vi "SL_Facade.vi"(0 "Data In":T4, 2 "Display State In":T2, 3 "Container State":T3) -> (6 "Data Out":T4, 7 "Display State Out":T2, 8 "Action":T1)   [LabVIEW 2020, in "SL_XControl.xctl"]
uses:
  SL_XControl.xctl
  SL_Data.ctl
  <vilib>/_xctls/Container State.ctl
  SL_State.ctl
  <vilib>/_xctls/Action.ctl
  <vilib>/_xctls/XControlSupport.lvlib
panel:
  out "type":string
  out "value":string
  out "Toggle":bool
  out "info":string
  in  "Refresh":bool
  in  "Login":bool
  in  "Edit":bool
  in  "Property":string
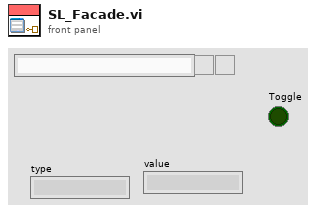
[diagram p1: front panel]
types:
  T1 = typedef "XControlSupport.lvlib/Action.ctl" = cluster{"Data Changed?":bool, "State Changed?":bool, "Action Name":string}
  T2 = typedef "SL_XControl.xctl/SL_State.ctl" = cluster{"Numeric":dbl}
  T3 = typedef "XControlSupport.lvlib/Container State.ctl" = cluster{"Indicator?":bool, "Run Mode?":bool, " Refnum":refnum<vi>}
  T4 = typedef "SL_XControl.xctl/SL_Data.ctl" = string
  T5 = enum8{"Enabled", "Disabled", "Disabled and Grayed Out"}
  T6 = cluster{"Name":string, "BaseURL":string, "AppKey":string, "Headers":string[], "Timeout":i32}
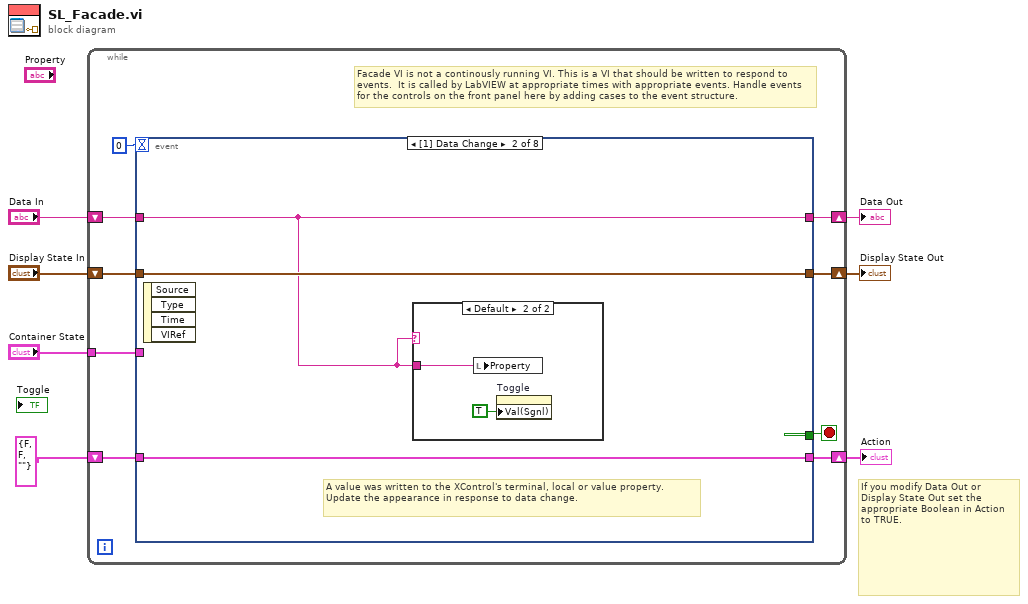
[diagram p0: block diagram]
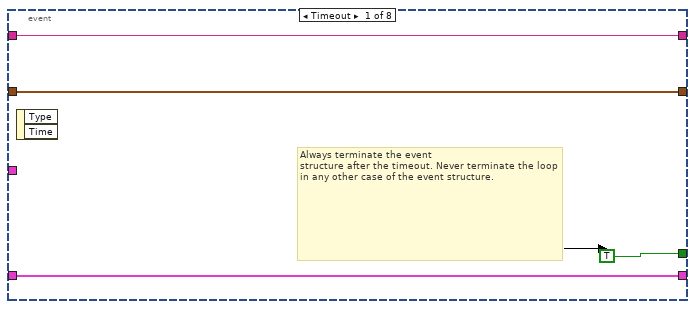
[diagram p2: hidden frame]
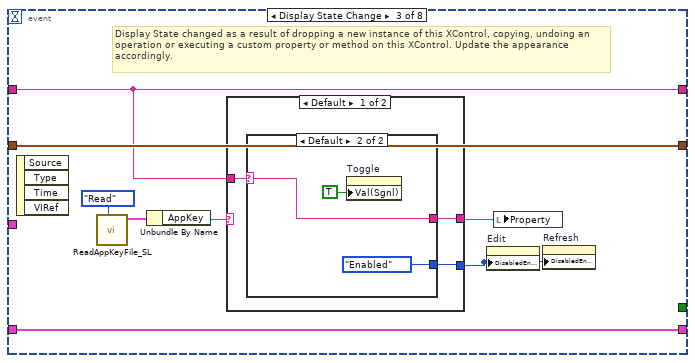
[diagram p4: hidden frame]
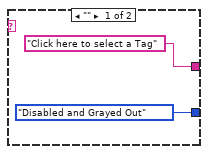
[diagram p5: hidden frame]
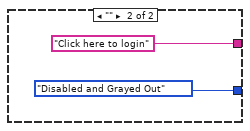
[diagram p6: hidden frame]
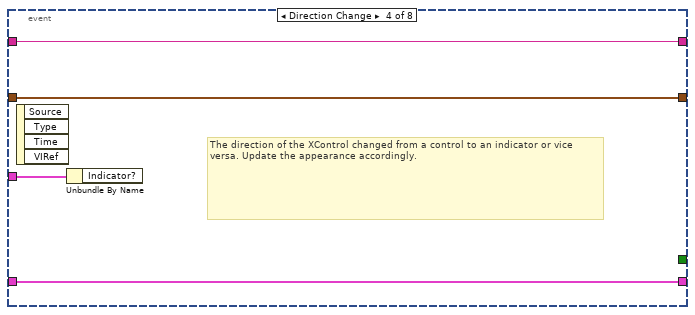
[diagram p7: hidden frame]
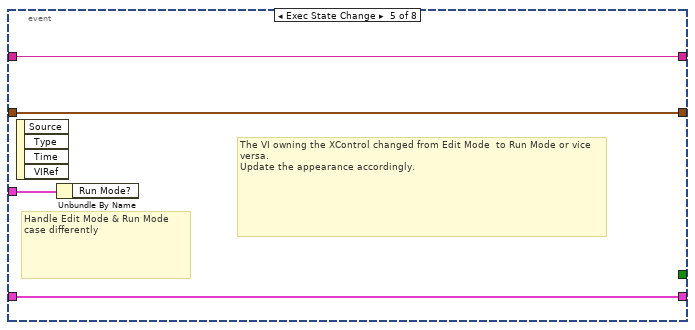
[diagram p8: hidden frame]
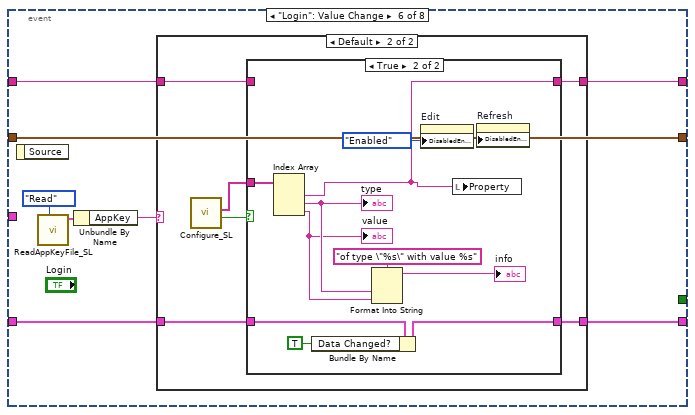
[diagram p9: hidden frame]
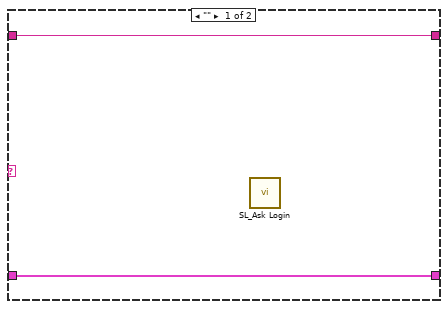
[diagram p10: hidden frame]
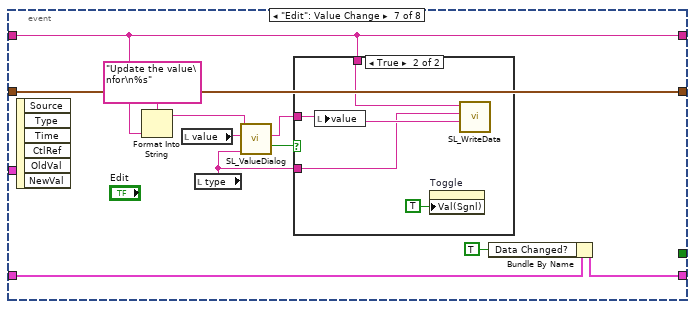
[diagram p12: hidden frame]
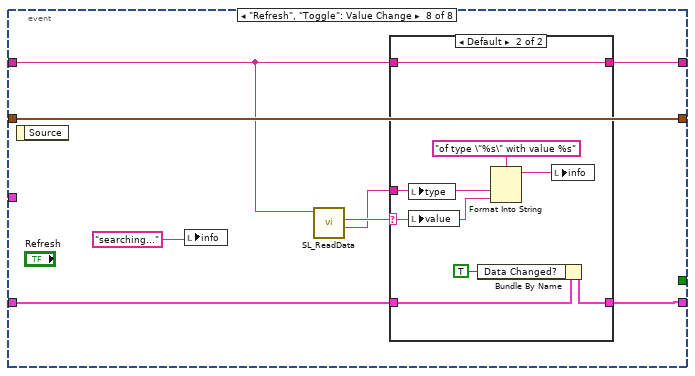
[diagram p14: hidden frame]
diagram:
  # "If you modify Data Out or\nDisplay State Out set the\nappropriate Boolean in Action\nto TRUE."
  n1 = while {
    shift-right: [w15] -> w4
    shift-left: "Display State In" -> [w16]
    tunnel: "Container State" -> [w12]
    shift-right: [w10] -> w7
    shift-left: "Data In" -> [w11]
    shift-right: [w8] -> w2
    shift-left: T1 {"Data Changed?"=FALSE, "State Changed?"=FALSE, "Action Name"=""} ("Action") -> [w9]
    stop <- w14 stop-if-true
    # "Facade VI is not a continously running VI. This is a VI that should be written to respond to events.  It is called by LabVIEW at appropriate times with appropriate events. Handle events for the controls on the front panel here by adding cases to the event structure."
    n2 = event shown="[1] Data Change" {
      selector: _ -> [_ _ _ _ _ _ _ _]
      dyn-events: _ -> [_ _ _ _ _ _ _ _]
      timeout: 0 -> [_ _ _ _ _ _ _ _]
      tunnel: w16 -> [w18 w23 w33 w46 w50 w59 w90 w102]
      tunnel: [w18 w23 w33 w46 w50 w59 w90 w102] -> w15
      tunnel: [TRUE _ _ _ _ _ _ _] -> w14
      tunnel: w12 -> [_ _ _ w47 w51 _ _ _]
      tunnel: w11 -> [w17 w21 w26 w45 w49 w56 w85 w95]
      tunnel: [w17 w21 w26 w45 w49 w55 w85 w101] -> w10
      tunnel: [w19 w22 w32 w44 w48 w57 w81 w99] -> w8
      tunnel: w9 -> [w19 w22 w32 w44 w48 w58 w82 w100]
      event Timeout {
        # "Always terminate the event\nstructure after the timeout. Never terminate the loop in any other case of the event structure."
        n3 = event-data() -> ()  [unwired: 1 in, 2 out]
      }
      event Data Change {
        # "A value was written to the XControl's terminal, local or value property.\nUpdate the appearance in response to data change."
        n4 = event-data() -> ()  [unwired: 1 in, 4 out]
        n5 = case shown="Default" w21 {
          tunnel: w21 -> [_ w24]
          frame "" {
          }
          frame Default {
            n6 = local write "Property"(w24) -> ()
            n7 = property on="Toggle" class="Bool (strict)"("Val(Sgnl)"=TRUE ("Value (Signaling)")) -> ()  [unwired: 2 in, 2 out]
          }
        }
      }
      event Display State Change {
        # "Display State changed as a result of dropping a new instance of this XControl, copying, undoing an operation or executing a custom property or method on this XControl. Update the appearance accordingly."
        n8 = event-data() -> ()  [unwired: 1 in, 4 out]
        n9 = call "ReadAppKeyFile_SL.vi"("Task"=enum16{"Read", "Write"}."Read") -> ("Device Out"=w31:T6)  [unwired: 8 in, 2 out]
        n10 = Unbundle By Name(w31) -> ("AppKey"=w30:string)
        n11 = case shown="Default" w30 {
          tunnel: [w36 "Click here to login" ("Property")] -> w29
          tunnel: [w35 T5."Disabled and Grayed Out" ("Disabled")] -> w28
          tunnel: w26 -> [w34 _]
          frame Default {
            n12 = case shown="Default" w34 {
              selector: w34 -> [_ w39]
              tunnel: ["Click here to select a Tag" ("Property") w39] -> w36
              tunnel: [T5."Disabled and Grayed Out" ("Disabled") T5."Enabled" ("Disabled")] -> w35
              frame "" {
              }
              frame Default {
                n13 = property on="Toggle" class="Bool (strict)"("Val(Sgnl)"=TRUE ("Value (Signaling)")) -> ()  [unwired: 2 in, 2 out]
              }
            }
          }
          frame "" {
          }
        }
        n14 = property on="Edit" class="Bool"("DisabledEnum"=w28) -> ()  [unwired: 2 in, 2 out]
        n15 = local write "Property"(w29) -> ()
        n16 = property on="Refresh" class="Bool"("DisabledEnum"=w28) -> ()  [unwired: 2 in, 2 out]
      }
      event Direction Change {
        # "The direction of the XControl changed from a control to an indicator or vice versa. Update the appearance accordingly."
        n17 = event-data() -> ()  [unwired: 1 in, 4 out]
        n18 = Unbundle By Name(w47) -> ()  [unwired: 1 out]
      }
      event Exec State Change {
        # "The VI owning the XControl changed from Edit Mode  to Run Mode or vice versa.\nUpdate the appearance accordingly."
        # "Handle Edit Mode & Run Mode\ncase differently"
        n19 = event-data() -> ()  [unwired: 1 in, 4 out]
        n20 = Unbundle By Name(w51) -> ()  [unwired: 1 out]
      }
      event "Login": Value Change {
        n21 = event-data() -> ()  [unwired: 1 in, 1 out]
        n22 = call "ReadAppKeyFile_SL.vi"("Task"=enum16{"Read", "Write"}."Read") -> ("Device Out"=w54:T6)  [unwired: 8 in, 2 out]
        n23 = Unbundle By Name(w54) -> ("AppKey"=w52:string)
        n24 = case shown="Default" w52 {
          tunnel: w58 -> [w60 w67]
          tunnel: [w60 w66] -> w57
          tunnel: w56 -> [w61 w65]
          tunnel: [w61 w64] -> w55
          frame "" {
            n25 = call "SL_Ask Login.vi"() -> ()  [unwired: 10 in, 2 out]
          }
          frame Default {
            n26 = call "Configure_SL.vi"() -> ("changed?"=w63:bool, "Property"=w62:string[])  [unwired: 10 in]
            n27 = case shown="True" w63 {
              tunnel: w65 -> [w69 _]
              tunnel: [w69 w72] -> w64
              tunnel: w62 -> [_ w79]
              tunnel: w67 -> [w68 w77]
              tunnel: [w68 w76] -> w66
              frame False {
              }
              frame True {
                w73 = T5."Enabled" ("Disabled")
                n28 = Index Array(array=w79) -> (element #1=w72:string, element #2=w71:string, element #3=w70:string)  [unwired: 3 in]
                "value" <- w70
                "type" <- w71
                n29 = Bundle By Name(cluster=w77, "Data Changed?"=TRUE) -> (w76:T1)
                n30 = Format Into String(format string="of type \"%s\" with value %s", w71, w70) -> (resulting string=→"info":string)  [unwired: 2 in, 1 out]
                n31 = property on="Edit" class="Bool"("DisabledEnum"=w73) -> ()  [unwired: 2 in, 2 out]
                n32 = local write "Property"(w72) -> ()
                n33 = property on="Refresh" class="Bool"("DisabledEnum"=w73) -> ()  [unwired: 2 in, 2 out]
              }
            }
          }
        }
      }
      event "Edit": Value Change {
        n34 = event-data() -> ()  [unwired: 1 in, 6 out]
        n35 = Format Into String(format string="Update the value\nfor\n%s", w85) -> (resulting string=w86:string)  [unwired: 2 in, 1 out]
        n36 = local read "value"() -> (w84:string)
        n37 = local read "type"() -> (w80:string)
        n38 = call "SL_ValueDialog.vi"("type"=w80, "Value"=w84, "Title"=w86) -> ("replace?"=w89:bool, "Value out"=w88:string)  [unwired: 7 in]
        n39 = case shown="True" w89 {
          tunnel: w85 -> [_ w93]
          tunnel: w88 -> [_ w92]
          tunnel: w80 -> [_ w91]
          frame False {
          }
          frame True {
            n40 = local write "value"(w92) -> ()
            n41 = property on="Toggle" class="Bool (strict)"("Val(Sgnl)"=TRUE ("Value (Signaling)")) -> ()  [unwired: 2 in, 2 out]
            n42 = call "SL_WriteData.vi"("Data"=w92, "Type"=w91, "Path"=w93) -> ()  [unwired: 9 in]
          }
        }
        n43 = Bundle By Name(cluster=w82, "Data Changed?"=TRUE) -> (w81:T1)
      }
      event "Refresh", "Toggle": Value Change {
        n44 = event-data() -> ()  [unwired: 1 in, 1 out]
        n45 = local write "info"("searching..." ("info")) -> ()
        n46 = call "SL_ReadData.vi"("Property"=w95) -> ("type"=w97:string, "value"=w98:string)  [unwired: 9 in]
        n47 = case shown="Default" w98 {
          selector: w98 -> [_ w106]
          tunnel: w95 -> [w104 w107]
          tunnel: [w104 w107] -> w101
          tunnel: w100 -> [w103 w112]
          tunnel: [w103 w111] -> w99
          tunnel: w97 -> [_ w105]
          frame "" {
          }
          frame Default {
            n48 = local write "type"(w105) -> ()
            n49 = local write "value"(w106) -> ()
            n50 = Bundle By Name(cluster=w112, "Data Changed?"=TRUE) -> (w111:T1)
            n51 = Format Into String(format string="of type \"%s\" with value %s", w105, w106) -> (resulting string=w108:string)  [unwired: 2 in, 1 out]
            n52 = local write "info"(w108) -> ()
          }
        }
      }
    }
  }
  "Display State Out" <- w4
  "Data Out" <- w7
  "Action" <- w2
